vi "Modify Dequeue Cmds to Requested Node Size.vi"(7 "VI to Code Relative Path":string="IONode\\DLULayer\\Dequeue Cmds From Nodes.vi", 8 "Error In":errorcluster, 10 "NumCases":i32=1, 11 "Source Root Path":path=path "C:/Users/kvemishe/Downloads/IONode/DLULayer/Dequeue Cmds From Nodes.vi") -> (0 "Error Out":errorcluster, 1 "Found Object?":bool, 3 "Source Root Path Out":path=path "C:/Users/kvemishe/Downloads/IONode/DLULayer/Dequeue Cmds From Nodes.vi")   [LabVIEW 2014]
doc: "This VI is made to script the SPI Engine \"Dequeue Cmds from Nodes\" and \"Enqueue Data to Nodes\" VI. In each VI, it duplicates a case structure and selects the appropriate FIFO name to allow the engine to retrieve the data acquiried by every Data Node. One case structure should be created for every Data Node in the engine. There should be one Data Node for every channel on the bus."
uses:
  <vilib>/Utility/traverseref.llb/TRef TravTarget.ctl
  <vilib>/Utility/traverseref.llb/VI Scripting - Traverse.lvlib
  Initialization Scripting/SPI Engine Scripting.lvlib
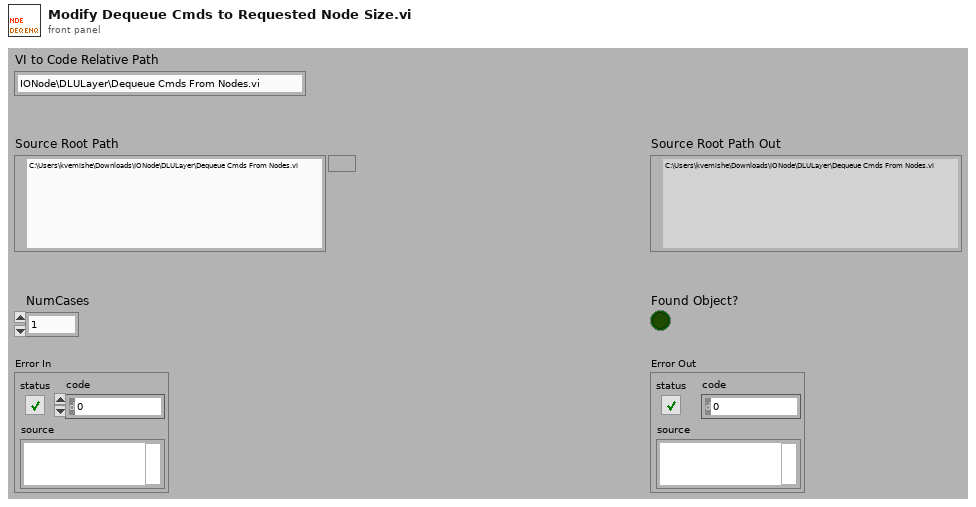
[diagram p1: front panel]
types:
  T1 = typedef "TRef TravTarget.ctl" = enum16{"FP", "BD", "Other"}
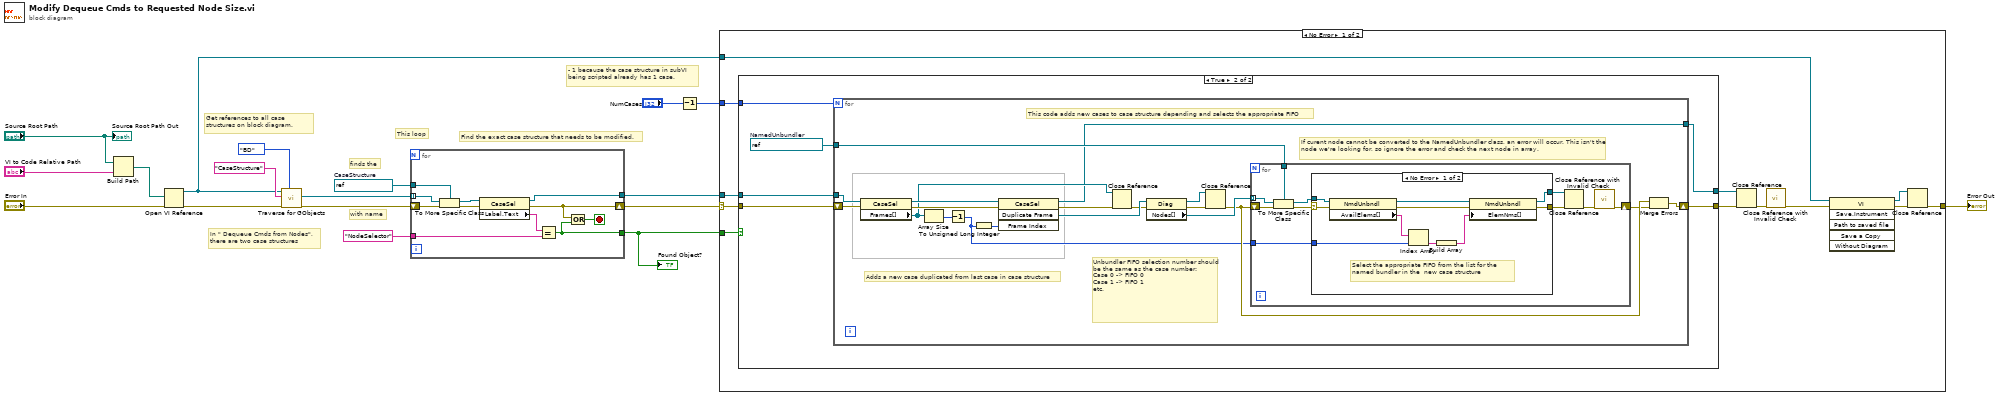
[diagram p0: block diagram]
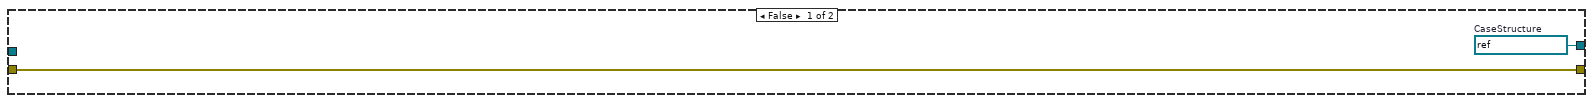
[diagram p2: hidden frame]
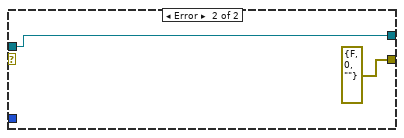
[diagram p3: hidden frame]
diagram:
  w3 = refnum<vi> refnum  # CaseStructure
  # "- 1 because the case structure in subVI being scripted already has 1 case."
  # "Find the exact case structure that needs to be modified."
  # "This loop"
  # "Get references to all case structures on block diagram."
  # "finds the"
  # "with name"
  # "In \" Dequeue Cmds from Nodes\",\nthere are two case structures"
  n1 = Build Path(base path="Source Root Path", name or relative path="VI to Code Relative Path") -> (appended path=w7:path)
  n2 = Open VI Reference(vi path=w7, error in (no error)="Error In") -> (vi reference=w10:refnum<vi>, error out=w17:errorcluster)  [unwired: 4 in]
  n3 = call <vilib>:"Traverse for GObjects.vi"("Traverse Target"=TRef_TravTarget."BD", "error in (no error)"=w17, "Class Name"="CaseStructure", "VI Refnum"=w10) -> ("error out"=w14:errorcluster, "References"=w15:refnum<vi>[])  [unwired: 4 in, 2 out]
  n4 = for {
    tunnel: w15 -> [w29] mode=indexing
    shift-right: [w24] -> w12
    shift-left: w14 -> [w28]
    tunnel: [w23] -> w11
    tunnel: [w22] -> w13
    tunnel: "NodeSelector" ("y") -> [w20]
    tunnel: w3 -> [w21]
    stop <- w25 stop-if-true
    n5 = To More Specific Class(target class=w21, reference=w29, error in=w28) -> (specific class reference=w27:refnum<vi>, error out=w26:errorcluster)
    n6 = property class="CaseSel"(reference=w27, error in=w26) -> (reference out=w22:refnum<vi>, error out=w24:errorcluster, "Label.Text"=w19:string)
    n7 = Equal?(x=w19, y=w20) -> (x = y?=w23:bool)
    n8 = Or(x=w24, y=w23) -> (x .or. y?=w25:bool)
  }
  "Found Object?" <- w11
  n9 = Decrement(x="NumCases") -> (x-1=w1:i32)
  n10 = case shown="No Error" w12 {
    selector: w12 -> [w39 w91]
    tunnel: w13 -> [w41 _]
    tunnel: w11 -> [w40 _]
    tunnel: w1 -> [w34 _]
    tunnel: w10 -> [w36 _]
    tunnel: [w35 w91] -> w8
    frame No Error {
      n11 = case shown="True" w40 {
        tunnel: w41 -> [_ w49]
        tunnel: w39 -> [w43 w48]
        tunnel: [w43 w47] -> w33
        tunnel: w34 -> [_ w45]
        tunnel: [w42 w44] -> w32
        frame False {
          w42 = refnum<vi> refnum  # CaseStructure
        }
        frame True {
          w46 = refnum<vi> refnum  # NamedUnbundler
          n12 = for {
            N: w45 -> [_]
            tunnel: w49 -> [w63]
            shift-right: [w61] -> w47
            shift-left: w48 -> [w62]
            tunnel: w46 -> [w60]
            tunnel: [w50] -> w44
            # "If curent node cannot be converted to the NamedUnbundler class, an error will occur. This isn't the node we're looking for, so ignore the error and check the next node in array."
            # "Unbundler FIFO selection number should be the same as the case number:\nCase 0 -> FIFO 0\nCase 1 -> FIFO 1\netc."
            # "Adds a new case duplicated from last case in case structure"
            # "This code adds new cases to case structure depending and selects the appropriate FIFO"
            n13 = property class="CaseSel"(reference=w63, error in=w62) -> (reference out=w68:refnum<vi>, error out=w67:errorcluster, "Frames[]"=w59:refnum<vi>[])
            n14 = Array Size(array=w59) -> (size(s)=w66:i32)
            n15 = Decrement(x=w66) -> (x-1=w53:i32)
            n16 = To Unsigned Long Integer(number=w53) -> (unsigned 32bit integer=w52:u32)
            n17 = invoke class="CaseSel" method="Duplicate Frame"(reference=w68, error in=w67, "Frame Index"=w52) -> (reference out=w50:refnum<vi>, error out=w51:errorcluster, "Duplicate Frame"=w65:refnum<vi>)  [unwired: 1 in, 1 out]
            n18 = Close Reference(reference=w59, error in (no error)=w51) -> (error out=w58:errorcluster)
            n19 = property class="Diag"(reference=w65, error in=w58) -> (reference out=w56:refnum<vi>, error out=w57:errorcluster, "Nodes[]"=w64:refnum<vi>[])
            n20 = Close Reference(reference=w56, error in (no error)=w57) -> (error out=w55:errorcluster)
            n21 = for {
              tunnel: w64 -> [w78] mode=indexing
              tunnel: w60 -> [w77]
              tunnel: w53 -> [w74]
              shift-right: [w72] -> w54
              shift-left: w55 -> [w73]
              n22 = To More Specific Class(target class=w77, reference=w78, error in=w73) -> (specific class reference=w75:refnum<vi>, error out=w76:errorcluster)
              n23 = case shown="No Error" w76 {
                selector: w76 -> [w87 _]
                tunnel: w75 -> [w88 w89]
                tunnel: w74 -> [w82 _]
                tunnel: [w80 errorcluster {"status"=FALSE, "code"=0, "source"=""} ("error out")] -> w71
                tunnel: [w79 w89] -> w70
                frame No Error {
                  # "Select the appropriate FIFO from the list for the named bundler in the  new case structure"
                  n24 = property class="NmdUnbndl"(reference=w88, error in=w87) -> (reference out=w86:refnum<vi>, error out=w81:errorcluster, "AvailElems[]"=w85:string[])
                  n25 = Index Array(array=w85, index=w82) -> (element=w84:string)
                  n26 = Build Array(w84) -> (w83:string[])
                  n27 = property class="NmdUnbndl"(reference=w86, error in=w81, "ElemNms[]"=w83) -> (reference out=w79:refnum<vi>, error out=w80:errorcluster)
                }
                frame Error {
                }
              }
              n28 = Close Reference(reference=w70, error in (no error)=w71) -> (error out=w69:errorcluster)
              n29 = call "Close Reference with Invalid Check.vi"("error in (no error)"=w69) -> ("error out"=w72:errorcluster)  [unwired: 10 in]
            }
            n30 = Merge Errors(w55, w54) -> (w61:errorcluster)
          }
        }
      }
      n31 = Close Reference(reference=w32, error in (no error)=w33) -> (error out=w31:errorcluster)
      n32 = call "Close Reference with Invalid Check.vi"("error in (no error)"=w31) -> ("error out"=w30:errorcluster)  [unwired: 10 in]
      n33 = invoke class="VI" method="Save.Instrument"(reference=w36, error in=w30) -> (reference out=w38:refnum<vi>, error out=w37:errorcluster)  [unwired: 4 in, 4 out]
      n34 = Close Reference(reference=w38, error in (no error)=w37) -> (error out=w35:errorcluster)
    }
    frame Error {
    }
  }
  "Error Out" <- w8
  "Source Root Path Out" <- "Source Root Path"
